vi "lab10_target_2.vi"() -> ()   [LabVIEW 2020]
uses:
  <vilib>/Platform/TimedLoop/XDataNode/timing_clust.ctl
  <vilib>/Platform/TimedLoop/XDataNode/nitl_modes.ctl
  <vilib>/Platform/TimedLoop/XDataNode/wakeup.ctl
  <vilib>/Platform/TimedLoop/scheduler/LVUserAPI/_suppVIs/Create_1MHz_TSource.vi
  <vilib>/platform/TimedLoop/XDataNode/XDataNode.xnode
  <vilib>/Platform/TimedLoop/XDataNode/XDNodeRunTimeDep.lvlib
panel:
  out "start_time":dbl
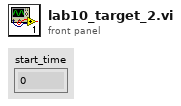
[diagram p1: front panel]
types:
  T1 = typedef "XDNodeRunTimeDep.lvlib/timing_clust.ctl" = cluster{"Expected End [f-1]":u64, "Actual End [f-1]":u64, "Finished Late? [f-1]":bool, "Expected End [i-1]":u64, "Actual End [i-1]":u64, "Finished Late? [i-1]":bool, "Expected Start [i]":u64, "Actual Start [i]":u64, "Expected Start [f]":u64, "Actual Start [f]":u64, "Source Name":string, "Structure Name":string, "Period":i64, "Deadline":i64, "Offset":i64, "Start":i64, "Priority":i32, "Timeout":i32, "Mode":T2, "Wakeup Reason":T3, "Error":errorcluster, "Source Type":string, "Secondary Source Type":string, "Global End Time":u64, "Global Start Time":u64, "Frame Duration":u64, "Iteration Duration":u64, "Assigned CPU":i32, "I/O Scan Engine Mode":u32}
  T2 = typedef "XDNodeRunTimeDep.lvlib/nitl_modes.ctl" = enum32{"No Change", "Process missed periods, maintain original phase", "Discard missed periods, maintain original phase", "Process missed periods, ignore original phase", "Discard missed periods, ignore original phase"}
  T3 = typedef "XDNodeRunTimeDep.lvlib/wakeup.ctl" = enum32{"Normal", "Aborted", "Asynchronous wakeup", "Timing source error", "Timed loop error", "Timeout"}
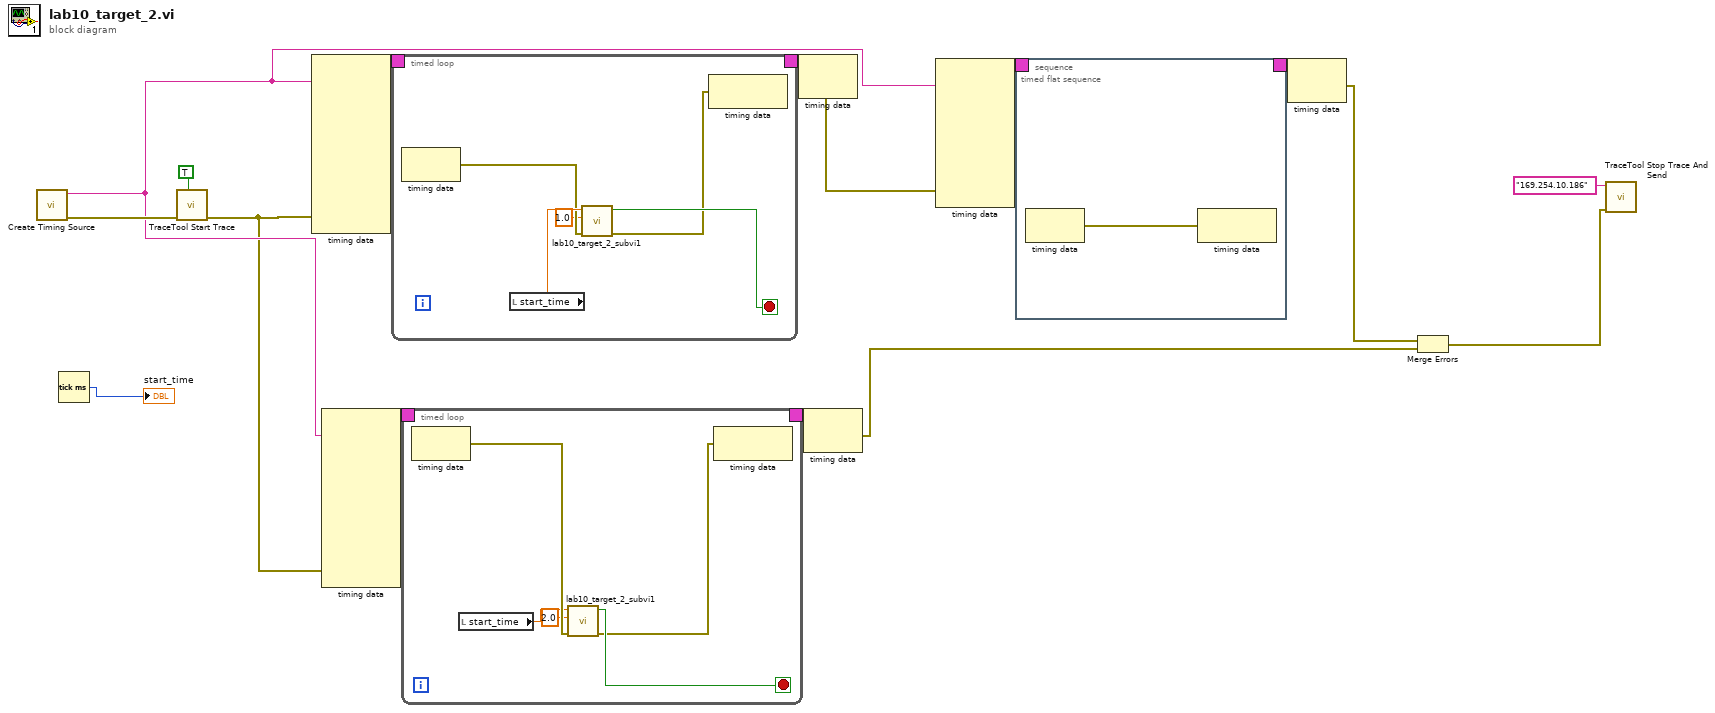
[diagram p0: block diagram]
diagram:
  n1 = call-poly <vilib>:"Create Timing Source.vi"() -> ("error out"=w11:errorcluster, "name (out)"=w5:string)  [unwired: 10 in]
  n2 = Tick Count (ms)() -> (millisecond timer value=→"start_time":u32)
  n3 = call <vilib>:"TraceTool Start Trace.vi"("Detailed Tracing? (F)"=TRUE, "error in (no error)"=w11) -> ("error out"=w1:errorcluster)  [unwired: 8 in, 1 out]
  n4 = node-c288(w5, w1) -> (w16:T1)  [unwired: 8 in]
  n5 = node-c288(w5, w1) -> (w7:T1)  [unwired: 8 in]
  n6 = timed-loop {
    timing: w16 -> [_]
    timing-out: [_] -> w15
    stop <- w20 stop-if-true
    n7 = node-c288() -> (w19:errorcluster)  [unwired: 1 in]
    n8 = local read "start_time"() -> (w21:dbl)
    n9 = call "lab10_target_2_subvi1.vi"("error in (no error)"=w19, "event_id"=1.0, "start_time"=w21) -> ("error out"=w18:errorcluster, "Boolean"=w20:bool)  [unwired: 7 in]
    n10 = node-c288(w18) -> ()  [unwired: 1 out]
  }
  n11 = timed-loop {
    timing: w7 -> [_]
    timing-out: [_] -> w6
    stop <- w31 stop-if-true
    n12 = node-c288() -> (w29:errorcluster)  [unwired: 1 in]
    n13 = local read "start_time"() -> (w28:dbl)
    n14 = call "lab10_target_2_subvi1.vi"("error in (no error)"=w29, "event_id"=2.0, "start_time"=w28) -> ("error out"=w30:errorcluster, "Boolean"=w31:bool)  [unwired: 7 in]
    n15 = node-c288(w30) -> ()  [unwired: 1 out]
  }
  n16 = node-c288(w15) -> (w12:errorcluster)
  n17 = node-c288(w6) -> (w4:errorcluster)
  n18 = node-c288(w5, w12) -> (w14:T1)  [unwired: 6 in]
  n19 = timed-sequence {
    timing: w14 -> [_]
    timing-out: [_] -> w13
    n20 = timed-flat-sequence {
      n21 = node-c288() -> (w37:errorcluster)  [unwired: 1 in]
      n22 = node-c288(w37) -> ()  [unwired: 1 out]
    }
  }
  n23 = node-c288(w13) -> (w3:errorcluster)
  n24 = Merge Errors(w3, w4) -> (w2:errorcluster)
  n25 = call <vilib>:"TraceTool Stop Trace And Send.vi"("error in (no error)"=w2, "Trace Host Network Address"="169.254.10.186") -> ()  [unwired: 9 in, 1 out]
